vi "test all tethers.vi"(8 "error in":errorcluster, 11 "tether coords":dbl[][](array[numeric])) -> (0 "error out":errorcluster, 3 "tether coords out":dbl[][](array[numeric]))   [LabVIEW 2017]
uses:
  <vilib>/Utility/error.llb/DialogType.ctl
panel:
  out "resulting string":string
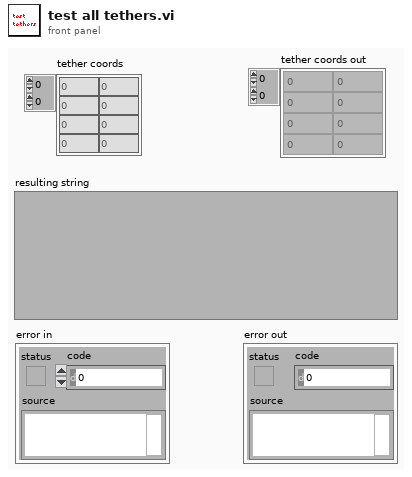
[diagram p1: front panel]
types:
  T1 = typedef "DialogType.ctl" = u16
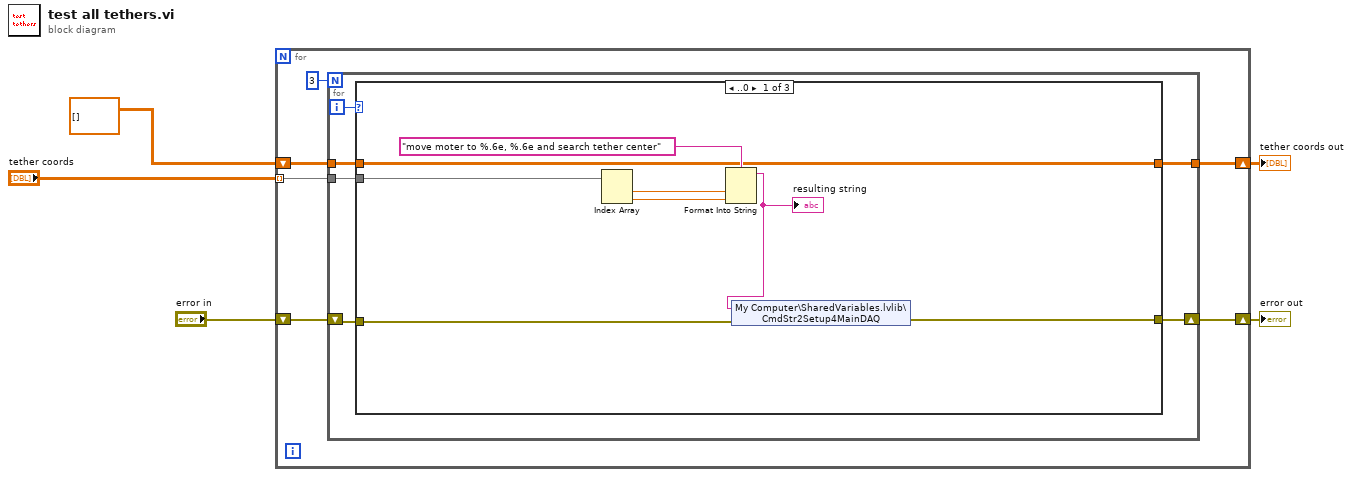
[diagram p0: block diagram]
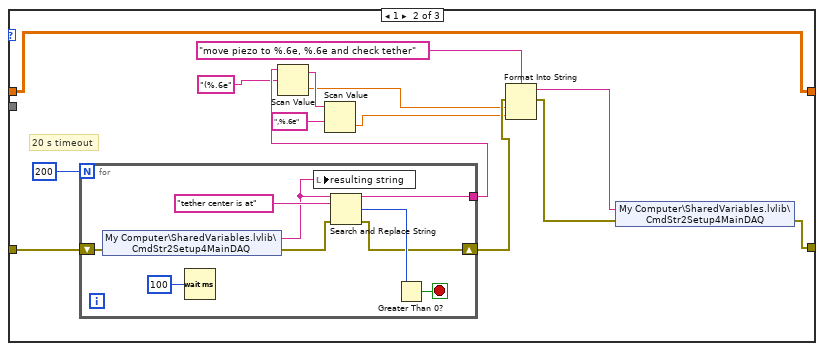
[diagram p2: hidden frame]
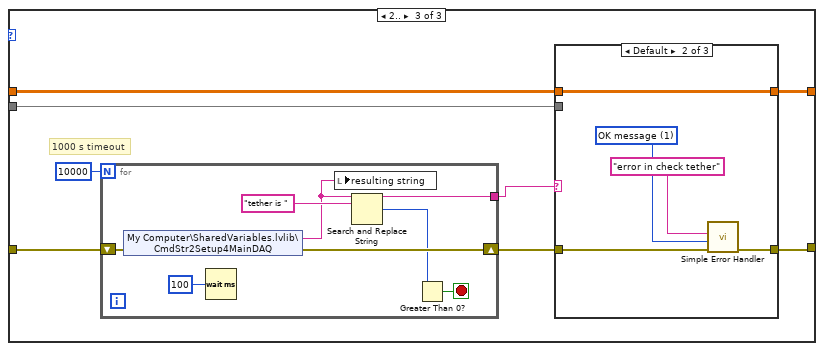
[diagram p3: hidden frame]
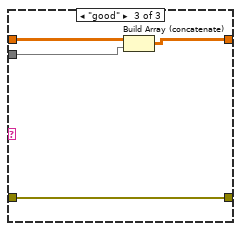
[diagram p5: hidden frame]
diagram:
  n1 = for {
    tunnel: "tether coords" -> [w11] mode=indexing
    shift-right: [w10] -> w3
    shift-left: "error in" -> [w9]
    shift-right: [w7] -> w2
    shift-left: dbl[][] [] -> [w8]
    n2 = for {
      N: 3 -> [_]
      tunnel: w11 -> [w17]
      tunnel: w8 -> [w14]
      tunnel: [w13] -> w7
      shift-right: [w16] -> w10
      shift-left: w9 -> [w15]
      i -> [w12]
      n3 = case shown="..0" w12 {
        tunnel: w17 -> [w25 _ w52]
        tunnel: [w19 w28 w49] -> w16
        tunnel: w15 -> [w21 w39 w56]
        tunnel: w14 -> [w18 w27 w51]
        tunnel: [w18 w27 w50] -> w13
        frame ..0 {
          n4 = Index Array(array=w25) -> (element #1=w24:dbl, element #2=w23:dbl)  [unwired: 2 in]
          n5 = Format Into String(format string="move moter to %.6e, %.6e and search tether center" ("CmdStr2Setup4MainDAQ"), w24, w23) -> (resulting string=w22:string)  [unwired: 2 in, 1 out]
          "resulting string" <- w22
          n6 = shared-variable "My Computer\\SharedVariables.lvlib\\CmdStr2Setup4MainDAQ"(w22, error in=w21) -> (error out=w19:errorcluster)
        }
        frame 1 {
          # "20 s timeout"
          n7 = for {
            N: 200 -> [_]
            shift-right: [w41] -> w35
            shift-left: w39 -> [w48]
            tunnel: [w44] -> w34
            stop <- w45 stop-if-true
            n8 = shared-variable "My Computer\\SharedVariables.lvlib\\CmdStr2Setup4MainDAQ"(error in=w48) -> (w40:string, error out=w42:errorcluster)
            n9 = Wait (ms)(milliseconds to wait=u32 100 ("millisecond multiple")) -> ()  [unwired: 1 out]
            n10 = local write "resulting string"(w40) -> ()
            n11 = Search and Replace String(input string=w40, search string="tether center is at", error in=w42) -> (result string=w44:string, number of replacements=w46:i32, error out=w41:errorcluster)  [unwired: 5 in, 1 out]
            n12 = Greater Than 0?(x=w46) -> (x > 0?=w45:bool)
          }
          n13 = Scan Value(string=w34, format string="(%.6e") -> (output string=w33:string, value=w31:dbl)  [unwired: 1 in]
          n14 = Scan Value(string=w33, format string=",%.6e") -> (value=w30:dbl)  [unwired: 1 in, 1 out]
          n15 = Format Into String(format string="move piezo to %.6e, %.6e and check tether" ("CmdStr2Setup4MainDAQ"), error in=w35, w31, w30) -> (resulting string=w26:string, error out=w36:errorcluster)  [unwired: 1 in]
          n16 = shared-variable "My Computer\\SharedVariables.lvlib\\CmdStr2Setup4MainDAQ"(w26, error in=w36) -> (error out=w28:errorcluster)
        }
        frame 2.. {
          # "1000 s timeout"
          n17 = for {
            N: 10000 -> [_]
            shift-right: [w74] -> w53
            shift-left: w56 -> [w75]
            tunnel: [w70] -> w54
            stop <- w71 stop-if-true
            n18 = shared-variable "My Computer\\SharedVariables.lvlib\\CmdStr2Setup4MainDAQ"(error in=w75) -> (w68:string, error out=w74:errorcluster)
            n19 = Wait (ms)(milliseconds to wait=u32 100 ("millisecond multiple")) -> ()  [unwired: 1 out]
            n20 = local write "resulting string"(w68) -> ()
            n21 = Search and Replace String(input string=w68, search string="tether is ") -> (result string=w70:string, number of replacements=w72:i32)  [unwired: 6 in, 2 out]
            n22 = Greater Than 0?(x=w72) -> (x > 0?=w71:bool)
          }
          n23 = case shown="Default" w54 {
            tunnel: w53 -> [w57 w63 w64]
            tunnel: [w57 w62 w64] -> w49
            tunnel: w52 -> [_ _ w67]
            tunnel: w51 -> [w58 w59 w66]
            tunnel: [w58 w59 w65] -> w50
            frame "bad" {
            }
            frame Default {
              (unwired) "" ("message")
              w61 = T1 1 items=["no dialog", "OK message", "continue or stop message", "OK message + warnings", "continue/stop + warnings"] ("type of dialog (OK msg:1)")
              n24 = call <vilib>:"Simple Error Handler.vi"("error source (\" \")"="error in check tether" ("search string"), "type of dialog (OK msg:1)"=w61, "error in (no error)"=w63) -> ("error out"=w62:errorcluster)  [unwired: 2 in, 4 out]
            }
            frame "good" {
              n25 = Build Array (concatenate)(w66, w67) -> (w65:dbl[][])
            }
          }
        }
      }
    }
  }
  "error out" <- w3
  "tether coords out" <- w2
